vi "Read Stop Notifier.vi"(11 "EMS Generic in":refnum<class "EMS Generic.lvclass">) -> (2 "stop":refnum<notifier>, 3 "EMS Generic out":refnum<class "EMS Generic.lvclass">)   [LabVIEW 2018, in "EMS Generic Actor.lvlib" / "EMS Generic.lvclass"]
uses:
  EMS Generic.lvclass
  EMS Generic.lvclass/EMS Generic.ctl
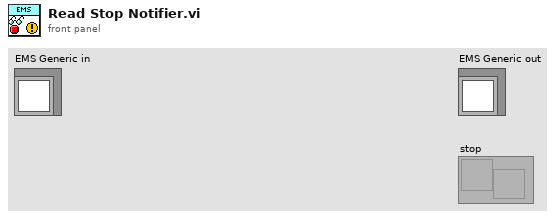
[diagram p1: front panel]
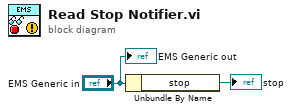
[diagram p0: block diagram]
diagram:
  n1 = Unbundle By Name("EMS Generic in") -> ("stop"=→"stop":refnum<notifier>)
  "EMS Generic out" <- "EMS Generic in"
